vi "autodrilling_V2.8 (DFT).vi"() -> ()   [LabVIEW 2011]
uses:
  <vilib>/DAQmx/write.llb/DAQmx Write (Digital Bool 1Line 1Point).vi
  <vilib>/DAQmx/create/channels.llb/DAQmx Create Channel (DO-Digital Output).vi
  <vilib>/DAQmx/miscellaneous.llb/DAQmx Fill In Error Info.vi
  <vilib>/Utility/file.llb/Write To Spreadsheet File (DBL).vi
panel:
  in  "stop":bool
  out "amplitude":dbl
  in  "number of samples":i32=15000
  out "row":i32
  out "column":i32
  in  "string":string="C:\\Users\\wired\\Desktop\\autodriller clone\\data\\20140624"
  out "depth":dbl
  in  "delta y":sgl=0.7
  in  "delta x":sgl=0.7
  in  "Number of rows (y)":sgl=2.0
  in  "Number of columns (x)":sgl=2.0
  out "origin y":sgl
  out "origin x":sgl
  out "origin z":sgl
  out "position y":sgl
  out "position x":sgl
  out "position z":sgl
  out "reference out 3":refnum<k7>
  in  "?":refnum<k7>(container)
  out "reference out 2":refnum<k7>
  in  "?":refnum<k7>(container)
  out "reference out":refnum<k7>
  in  "?":refnum<k7>(container)
  out "Waveform Graph":dynamicdata(graph)
  # "X"
  # "Z"
  # "Y"
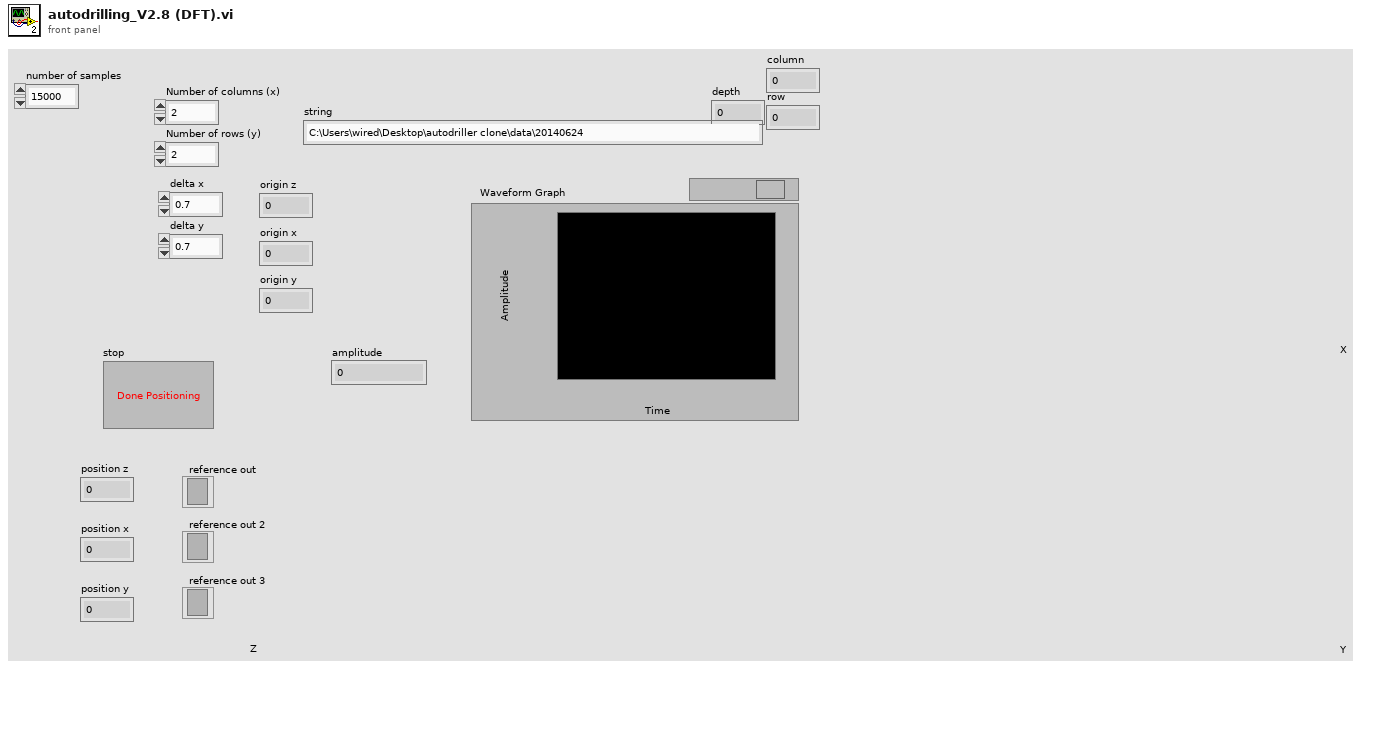
[diagram p1: front panel]
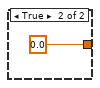
[diagram p2: hidden frame]
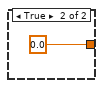
[diagram p3: hidden frame]
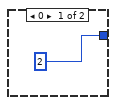
[diagram p4: hidden frame]
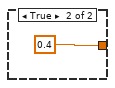
[diagram p5: hidden frame]
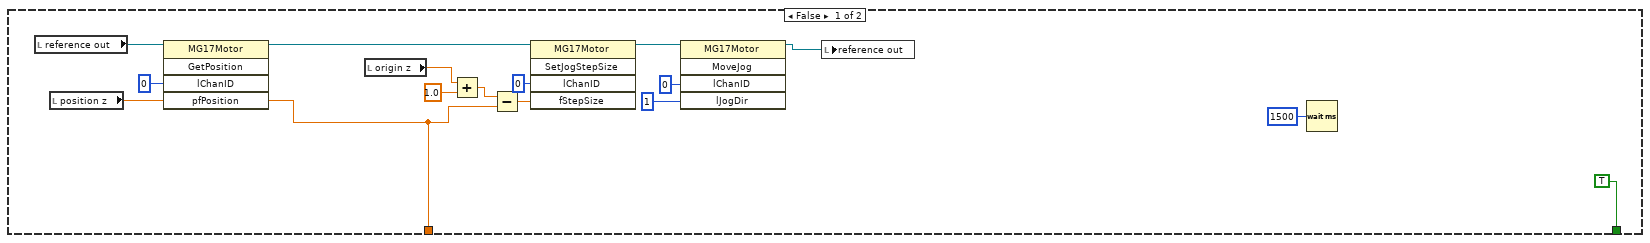
[diagram p6: hidden frame]
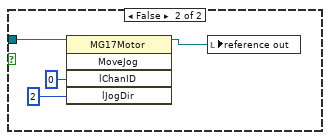
[diagram p7: hidden frame]
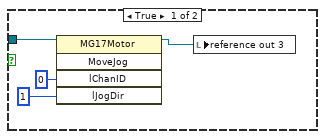
[diagram p8: hidden frame]
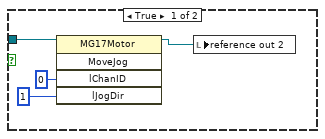
[diagram p9: hidden frame]
diagram:
  n1 = flat-sequence {
    frame #0 {
      # "move into position"
      n2 = property class="MG17Motor"(reference="?", "HWSerialNum"=83844140) -> (reference out=w9:refnum<k7>)  [unwired: 1 in, 1 out]
      n3 = property class="MG17Motor"(reference="?", "HWSerialNum"=83847372) -> (reference out=w6:refnum<k7>)  [unwired: 1 in, 1 out]
      n4 = property class="MG17Motor"(reference="?", "HWSerialNum"=83847391) -> (reference out=w12:refnum<k7>)  [unwired: 1 in, 1 out]
      n5 = invoke class="MG17Motor" method="StartCtrl"(reference=w9) -> (reference out=w2:refnum<k7>)  [unwired: 2 in, 2 out]
      n6 = invoke class="MG17Motor" method="StartCtrl"(reference=w6) -> (reference out=w1:refnum<k7>)  [unwired: 2 in, 2 out]
      n7 = invoke class="MG17Motor" method="StartCtrl"(reference=w12) -> (reference out=w3:refnum<k7>)  [unwired: 2 in, 2 out]
      n8 = while {
        tunnel: w3 -> [w30]
        tunnel: w2 -> [w29]
        tunnel: w1 -> [w28]
        stop <- "stop" stop-if-true
        n9 = local read "position z"() -> (w26:sgl)
        n10 = local read "position x"() -> (w23:sgl)
        n11 = local read "position y"() -> (w20:sgl)
        n12 = invoke class="MG17Motor" method="GetPosition"(reference=w30, "lChanID"=0, "pfPosition"=w26) -> (reference out=w27:refnum<k7>, "pfPosition"=w15:sgl)  [unwired: 2 in, 3 out]
        "position z" <- w15
        "origin z" <- w15
        n13 = invoke class="MG17Motor" method="GetPosition"(reference=w29, "lChanID"=0, "pfPosition"=w23) -> (reference out=w24:refnum<k7>, "pfPosition"=→"position x" →"origin x":sgl)  [unwired: 2 in, 3 out]
        n14 = invoke class="MG17Motor" method="GetPosition"(reference=w28, "lChanID"=0, "pfPosition"=w20) -> (reference out=w21:refnum<k7>, "pfPosition"=→"position y" →"origin y":sgl)  [unwired: 2 in, 3 out]
        n15 = local write "reference out 2"(w24) -> ()
        n16 = local write "reference out"(w27) -> ()
        n17 = local write "reference out 3"(w21) -> ()
        n18 = Subtract(x=w15, y=sgl 0.405) -> (x-y=→"depth":sgl)
      }
    }
    frame #1 {
      n19 = for {
        N: "Number of columns (x)" -> [_]
        tunnel: "Number of rows (y)" -> [w35]
        i -> [w33]
        n20 = flat-sequence {
          tunnel: [w48] -> w36
          tunnel: [w41] -> w34
          tunnel: w33 -> [w41]
          tunnel: w35 -> [w48]
          tunnel: w36 -> [w52]
          tunnel: w34 -> [w51]
          frame #0 {
            n21 = Equal?(x=0, y=w41) -> (x = y?=w37:bool)
            n22 = local read "reference out 2"() -> (w40:refnum<k7>)
            n23 = case shown="False" w37 {
              tunnel: [w49 0.0 ("y")] -> w38
              frame False {
                n24 = local read "delta x"() -> (w49:sgl)
              }
              frame True {
              }
            }
            n25 = invoke class="MG17Motor" method="SetJogStepSize"(reference=w40, "lChanID"=0, "fStepSize"=w38) -> (reference out=w43:refnum<k7>)  [unwired: 2 in, 4 out]
            n26 = invoke class="MG17Motor" method="MoveJog"(reference=w43, "lChanID"=0, "lJogDir"=2) -> (reference out=w44:refnum<k7>)  [unwired: 2 in, 4 out]
            n27 = Wait (ms)(milliseconds to wait=u32 4000) -> ()  [unwired: 1 out]
            n28 = local write "reference out 2"(w44) -> ()
          }
          frame #1 {
            n29 = for {
              N: w52 -> [_]
              tunnel: w51 -> [w55]
              i -> [w53]
              n30 = flat-sequence {
                tunnel: w55 -> [w66]
                tunnel: w53 -> [w61]
                tunnel: [w56] -> w54
                tunnel: w53 -> [w56]
                tunnel: w54 -> [w77]
                frame #0 {
                  n31 = Equal?(x=w61, y=0) -> (x = y?=w58:bool)
                  n32 = case shown="False" w58 {
                    tunnel: [w73 0.0 ("y")] -> w59
                    frame False {
                      n33 = local read "delta y"() -> (w73:sgl)
                    }
                    frame True {
                    }
                  }
                  n34 = local read "reference out 3"() -> (w57:refnum<k7>)
                  n35 = Add(x=w66, y=1.0) -> (x+y=w63:dbl)
                  n36 = invoke class="MG17Motor" method="SetJogStepSize"(reference=w57, "lChanID"=0, "fStepSize"=w59) -> (reference out=w70:refnum<k7>)  [unwired: 2 in, 4 out]
                  n37 = Quotient & Remainder(x=w63, y=2.0) -> (x-y*floor(x/y)=w64:dbl)  [unwired: 1 out]
                  n38 = case shown="1, Default" w64 {
                    tunnel: [2 ("lJogDir") 1 ("lJogDir")] -> w65
                    frame 0 {
                    }
                    frame 1, Default {
                    }
                  }
                  n39 = invoke class="MG17Motor" method="MoveJog"(reference=w70, "lChanID"=0, "lJogDir"=w65) -> (reference out=w69:refnum<k7>)  [unwired: 2 in, 4 out]
                  n40 = local write "reference out 3"(w69) -> ()
                  n41 = Wait (ms)(milliseconds to wait=u32 1500) -> ()  [unwired: 1 out]
                }
                frame #1 {
                  n42 = flat-sequence {
                    tunnel: w78 -> [w94]
                    frame #0 {
                      n43 = call-poly <vilib>:"DAQmx Create Virtual Channel.vi"("lines"=tag "Dev2/port0/line0") -> ("task out"=w83:refnum<k21>, "error out"=w84:errorcluster)  [unwired: 13 in]
                      n44 = call <vilib>:"DAQmx Start Task.vi"("task/channels in"=w83, "error in"=w84) -> ("task out"=w85:refnum<k21>, "error out"=w86:errorcluster)  [unwired: 12 in]
                      n45 = call-poly <vilib>:"DAQmx Write.vi"("task/channels in"=w85, "data"=TRUE, "error in"=w86) -> ("task out"=w87:refnum<k21>, "error out"=w88:errorcluster)  [unwired: 10 in, 1 out]
                      n46 = Wait (ms)(milliseconds to wait=u32 500) -> ()  [unwired: 1 out]
                      n47 = call <vilib>:"DAQmx Stop Task.vi"("task/channels in"=w87, "error in"=w88) -> ()  [unwired: 12 in, 2 out]
                    }
                    frame #1 {
                      n48 = local read "reference out"() -> (w97:refnum<k7>)
                      n49 = local read "position z"() -> (w103:sgl)
                      n50 = invoke class="MG17Motor" method="GetPosition"(reference=w97, "lChanID"=0, "pfPosition"=w103) -> (reference out=w99:refnum<k7>, "pfPosition"=w105:sgl)  [unwired: 2 in, 3 out]
                      n51 = local read "depth"() -> (w93:dbl)
                      n52 = Subtract(x=w105, y=w93) -> (x-y=w92:dbl)
                      n53 = Subtract(x=w92, y=w94) -> (x-y=w91:dbl)
                      n54 = invoke class="MG17Motor" method="SetJogStepSize"(reference=w99, "lChanID"=0, "fStepSize"=w91) -> (reference out=w100:refnum<k7>)  [unwired: 2 in, 4 out]
                      n55 = invoke class="MG17Motor" method="MoveJog"(reference=w100, "lChanID"=0, "lJogDir"=2) -> (reference out=w96:refnum<k7>)  [unwired: 2 in, 4 out]
                      n56 = local write "reference out"(w96) -> ()
                      n57 = Wait (ms)(milliseconds to wait=u32 2000) -> ()  [unwired: 1 out]
                    }
                    frame #2 {
                      n58 = call-poly <vilib>:"DAQmx Create Virtual Channel.vi"("lines"=tag "Dev2/port0/line0") -> ("task out"=w107:refnum<k21>, "error out"=w108:errorcluster)  [unwired: 13 in]
                      n59 = call <vilib>:"DAQmx Start Task.vi"("task/channels in"=w107, "error in"=w108) -> ("task out"=w109:refnum<k21>, "error out"=w110:errorcluster)  [unwired: 12 in]
                      n60 = call-poly <vilib>:"DAQmx Write.vi"("task/channels in"=w109, "data"=FALSE, "error in"=w110) -> ("task out"=w111:refnum<k21>, "error out"=w112:errorcluster)  [unwired: 10 in, 1 out]
                      n61 = Wait (ms)(milliseconds to wait=u32 4000) -> ()  [unwired: 1 out]
                      n62 = call <vilib>:"DAQmx Stop Task.vi"("task/channels in"=w111, "error in"=w112) -> ()  [unwired: 12 in, 2 out]
                    }
                  }
                  n63 = Equal To 0?(x=w77) -> (x = 0?=w79:bool)
                  n64 = case shown="False" w79 {
                    tunnel: [0.3 ("y") 0.4 ("y")] -> w78
                    frame False {
                    }
                    frame True {
                    }
                  }
                }
                frame #2 {
                  # "drill and record depth"
                  n65 = while {
                    tunnel: [w148] -> w126
                    tunnel: [w147] -> w120 mode=indexing
                    stop <- w149 stop-if-true
                    # "Im"
                    # "Re"
                    # "xn"
                    # "k"
                    n66 = Divide(x="number of samples", y=250.0 ("x")) -> (x/y=w135:dbl)
                    n67 = call "DAQ Assistant"("number of samples"="number of samples") -> ("data"=w146:dynamicdata)  [unwired: 16 in, 2 out]
                    "Waveform Graph" <- w146
                    n68 = call "Convert from Dynamic Data"("Dynamic Data Type"=w146) -> ("Array"=w133:dbl[])  [unwired: 3 in]
                    n69 = for {
                      N: "number of samples" -> [_]
                      tunnel: w133 -> [w157] mode=indexing
                      tunnel: w135 -> [w164]
                      tunnel: "number of samples" -> [w163]
                      shift-right: [w153] -> w138
                      shift-left: 0.0 -> [w155]
                      shift-right: [w150] -> w139
                      shift-left: 0.0 -> [w151]
                      i -> [w156]
                      # "val"
                      n70 = Divide(x=w156, y=w163) -> (x/y=w162:dbl)
                      n71 = Multiply(x=6.283185307179586, y=w164) -> (x*y=w161:dbl)
                      n72 = Multiply(x=w162, y=w161) -> (x*y=w160:dbl)
                      n73 = Sine(x=w160) -> (sin(x)=w158:dbl)
                      n74 = Cosine(x=w160) -> (cos(x)=w159:dbl)
                      n75 = Multiply(x=w157, y=w158) -> (x*y=w152:dbl)
                      n76 = Multiply(x=w157, y=w159) -> (x*y=w154:dbl)
                      n77 = Subtract(x=w151, y=w152) -> (x-y=w150:dbl)
                      n78 = Add(x=w155, y=w154) -> (x+y=w153:dbl)
                    }
                    n79 = Multiply(x=0.00047, y=0.65 ("threshold")) -> (x*y=w128:dbl)
                    n80 = Square(x=w139) -> (x^2=w142:dbl)
                    n81 = Square(x=w138) -> (x^2=w141:dbl)
                    n82 = Add(x=w141, y=w142) -> (x+y=w140:dbl)
                    n83 = Square Root(x=w140) -> (sqrt(x)=w143:dbl)
                    n84 = Divide(x=w143, y="number of samples") -> (x/y=w131:dbl)
                    n85 = Multiply(x=w131, y=2.0) -> (x*y=w130:dbl)
                    "amplitude" <- w130
                    n86 = Greater Or Equal?(x=w130, y=w128) -> (x >= y?=w145:bool)
                    n87 = case shown="True" w145 {
                      tunnel: [TRUE ("stop 2") FALSE ("stop 2")] -> w149
                      tunnel: [w170 _] -> w148
                      frame False {
                        n88 = local read "reference out"() -> (w173:refnum<k7>)
                        n89 = local read "position z"() -> (w180:sgl)
                        n90 = invoke class="MG17Motor" method="GetPosition"(reference=w173, "lChanID"=0, "pfPosition"=w180) -> (reference out=w176:refnum<k7>, "pfPosition"=w170:sgl)  [unwired: 2 in, 3 out]
                        n91 = local read "origin z"() -> (w166:sgl)
                        n92 = Add(x=w166, y=1.0) -> (x+y=w168:dbl)
                        n93 = Subtract(x=w168, y=w170) -> (x-y=w169:dbl)
                        n94 = invoke class="MG17Motor" method="SetJogStepSize"(reference=w176, "lChanID"=0, "fStepSize"=w169) -> (reference out=w177:refnum<k7>)  [unwired: 2 in, 4 out]
                        n95 = invoke class="MG17Motor" method="MoveJog"(reference=w177, "lChanID"=0, "lJogDir"=1) -> (reference out=w172:refnum<k7>)  [unwired: 2 in, 4 out]
                        n96 = local write "reference out"(w172) -> ()
                        n97 = Wait (ms)(milliseconds to wait=u32 1500) -> ()  [unwired: 1 out]
                      }
                      frame True {
                        n98 = flat-sequence {
                          frame #0 {
                            n99 = call-poly <vilib>:"DAQmx Create Virtual Channel.vi"("lines"=tag "Dev2/port0/line0") -> ("task out"=w184:refnum<k21>, "error out"=w185:errorcluster)  [unwired: 13 in]
                            n100 = call <vilib>:"DAQmx Start Task.vi"("task/channels in"=w184, "error in"=w185) -> ("task out"=w186:refnum<k21>, "error out"=w187:errorcluster)  [unwired: 12 in]
                            n101 = call-poly <vilib>:"DAQmx Write.vi"("task/channels in"=w186, "data"=TRUE, "error in"=w187) -> ("task out"=w188:refnum<k21>, "error out"=w189:errorcluster)  [unwired: 10 in, 1 out]
                            n102 = Wait (ms)(milliseconds to wait=u32 60) -> ()  [unwired: 1 out]
                            n103 = call <vilib>:"DAQmx Stop Task.vi"("task/channels in"=w188, "error in"=w189) -> ()  [unwired: 12 in, 2 out]
                          }
                          frame #1 {
                            n104 = local read "reference out"() -> (w192:refnum<k7>)
                            n105 = invoke class="MG17Motor" method="SetJogStepSize"(reference=w192, "lChanID"=0, "fStepSize"=sgl 0.005) -> (reference out=w196:refnum<k7>)  [unwired: 2 in, 4 out]
                            n106 = invoke class="MG17Motor" method="MoveJog"(reference=w196, "lChanID"=0, "lJogDir"=2) -> (reference out=w193:refnum<k7>)  [unwired: 2 in, 4 out]
                            n107 = Wait (ms)(milliseconds to wait=u32 100) -> ()  [unwired: 1 out]
                            n108 = local write "reference out"(w193) -> ()
                          }
                          frame #2 {
                            n109 = call-poly <vilib>:"DAQmx Create Virtual Channel.vi"("lines"=tag "Dev2/port0/line0") -> ("task out"=w201:refnum<k21>, "error out"=w202:errorcluster)  [unwired: 13 in]
                            n110 = call <vilib>:"DAQmx Start Task.vi"("task/channels in"=w201, "error in"=w202) -> ("task out"=w203:refnum<k21>, "error out"=w204:errorcluster)  [unwired: 12 in]
                            n111 = call-poly <vilib>:"DAQmx Write.vi"("task/channels in"=w203, "data"=FALSE, "error in"=w204) -> ("task out"=w205:refnum<k21>, "error out"=w206:errorcluster)  [unwired: 10 in, 1 out]
                            n112 = Wait (ms)(milliseconds to wait=u32 3500) -> ()  [unwired: 1 out]
                            n113 = call <vilib>:"DAQmx Stop Task.vi"("task/channels in"=w205, "error in"=w206) -> ()  [unwired: 12 in, 2 out]
                          }
                        }
                      }
                    }
                    n114 = Build Array(w148, w130) -> (w147:dbl[])
                  }
                  n115 = local read "column"() -> (w117:i32)
                  n116 = local write "depth"(w126) -> ()
                  n117 = local read "row"() -> (w116:i32)
                  n118 = Number To Decimal String(number=w117) -> (decimal integer string=w119:string)  [unwired: 1 in]
                  n119 = Number To Decimal String(number=w116) -> (decimal integer string=w118:string)  [unwired: 1 in]
                  n120 = Concatenate Strings("string", "_hole" ("string"), w119, w118, ".txt" ("string")) -> (w121:string)
                  n121 = String To Path(string=w121) -> (path=w125:path)
                  n122 = call-poly <vilib>:"Write To Spreadsheet File.vi"("format (%.3f)"="%e", "2D data"=w120, "file path (dialog if empty)"=w125) -> ()  [unwired: 5 in, 1 out]
                }
              }
              "row" <- w53
            }
          }
        }
        "column" <- w33
      }
    }
    frame #2 {
      n123 = Wait (ms)(milliseconds to wait=u32 2000) -> ()  [unwired: 1 out]
    }
    frame #3 {
      # "move to 0, 0.5, 0.5"
      n124 = local read "reference out"() -> (w212:refnum<k7>)
      n125 = local read "position z"() -> (w217:sgl)
      n126 = invoke class="MG17Motor" method="GetPosition"(reference=w212, "lChanID"=0, "pfPosition"=w217) -> (reference out=w215:refnum<k7>, "pfPosition"=w213:sgl)  [unwired: 2 in, 3 out]
      n127 = Subtract(x=sgl 25.0, y=w213) -> (x-y=w220:sgl)
      n128 = Absolute Value(x=w220) -> (abs(x)=w219:sgl)
      n129 = Greater Or Equal To 0?(x=w220) -> (x >= 0?=w221:bool)
      n130 = invoke class="MG17Motor" method="SetJogStepSize"(reference=w215, "lChanID"=0, "fStepSize"=w219) -> (reference out=w216:refnum<k7>)  [unwired: 2 in, 4 out]
      n131 = case shown="True" w221 {
        tunnel: w216 -> [w224 w228]
        frame True {
          n132 = invoke class="MG17Motor" method="MoveJog"(reference=w224, "lChanID"=0, "lJogDir"=1) -> (reference out=w225:refnum<k7>)  [unwired: 2 in, 4 out]
          n133 = local write "reference out"(w225) -> ()
        }
        frame False {
          n134 = invoke class="MG17Motor" method="MoveJog"(reference=w228, "lChanID"=0, "lJogDir"=2) -> (reference out=w229:refnum<k7>)  [unwired: 2 in, 4 out]
          n135 = local write "reference out"(w229) -> ()
        }
      }
      n136 = Wait (ms)(milliseconds to wait=u32 2000) -> ()  [unwired: 1 out]
    }
    frame #4 {
      w231 = sgl 6.25 ("x")
      n137 = local read "reference out 2"() -> (w250:refnum<k7>)
      n138 = local read "reference out 3"() -> (w240:refnum<k7>)
      n139 = local read "position x"() -> (w246:sgl)
      n140 = local read "position z"() -> (w236:sgl)
      n141 = invoke class="MG17Motor" method="GetPosition"(reference=w250, "lChanID"=0, "pfPosition"=w246) -> (reference out=w248:refnum<k7>, "pfPosition"=w251:sgl)  [unwired: 2 in, 3 out]
      n142 = invoke class="MG17Motor" method="GetPosition"(reference=w240, "lChanID"=0, "pfPosition"=w236) -> (reference out=w238:refnum<k7>, "pfPosition"=w241:sgl)  [unwired: 2 in, 3 out]
      n143 = Subtract(x=w231, y=w251) -> (x-y=w242:sgl)
      n144 = Subtract(x=w231, y=w241) -> (x-y=w232:sgl)
      n145 = Absolute Value(x=w242) -> (abs(x)=w244:sgl)
      n146 = Absolute Value(x=w232) -> (abs(x)=w234:sgl)
      n147 = Greater Or Equal To 0?(x=w242) -> (x >= 0?=w243:bool)
      n148 = Greater Or Equal To 0?(x=w232) -> (x >= 0?=w233:bool)
      n149 = invoke class="MG17Motor" method="SetJogStepSize"(reference=w248, "lChanID"=0, "fStepSize"=w244) -> (reference out=w247:refnum<k7>)  [unwired: 2 in, 4 out]
      n150 = invoke class="MG17Motor" method="SetJogStepSize"(reference=w238, "lChanID"=0, "fStepSize"=w234) -> (reference out=w237:refnum<k7>)  [unwired: 2 in, 4 out]
      n151 = case shown="False" w243 {
        tunnel: w247 -> [w262 w266]
        frame True {
          n152 = invoke class="MG17Motor" method="MoveJog"(reference=w262, "lChanID"=0, "lJogDir"=1) -> (reference out=w263:refnum<k7>)  [unwired: 2 in, 4 out]
          n153 = local write "reference out 2"(w263) -> ()
        }
        frame False {
          n154 = invoke class="MG17Motor" method="MoveJog"(reference=w266, "lChanID"=0, "lJogDir"=2) -> (reference out=w267:refnum<k7>)  [unwired: 2 in, 4 out]
          n155 = local write "reference out 2"(w267) -> ()
        }
      }
      n156 = case shown="False" w233 {
        tunnel: w237 -> [w254 w258]
        frame True {
          n157 = invoke class="MG17Motor" method="MoveJog"(reference=w254, "lChanID"=0, "lJogDir"=1) -> (reference out=w255:refnum<k7>)  [unwired: 2 in, 4 out]
          n158 = local write "reference out 3"(w255) -> ()
        }
        frame False {
          n159 = invoke class="MG17Motor" method="MoveJog"(reference=w258, "lChanID"=0, "lJogDir"=2) -> (reference out=w259:refnum<k7>)  [unwired: 2 in, 4 out]
          n160 = local write "reference out 3"(w259) -> ()
        }
      }
      n161 = Wait (ms)(milliseconds to wait=u32 5000) -> ()  [unwired: 1 out]
    }
    frame #5 {
      n162 = local read "reference out"() -> (w270:refnum<k7>)
      n163 = local read "reference out 2"() -> (w269:refnum<k7>)
      n164 = local read "reference out 3"() -> (w268:refnum<k7>)
      n165 = invoke class="MG17Motor" method="StopCtrl"(reference=w270) -> ()  [unwired: 2 in, 3 out]
      n166 = invoke class="MG17Motor" method="StopCtrl"(reference=w269) -> ()  [unwired: 2 in, 3 out]
      n167 = invoke class="MG17Motor" method="StopCtrl"(reference=w268) -> ()  [unwired: 2 in, 3 out]
    }
  }
